vi "Host - Alarm Init (SubVI).vi"(11 "GUI Data in":string[][](array[string])) -> (3 "Alarm Index":T1(array[cluster]))   [LabVIEW 2021]
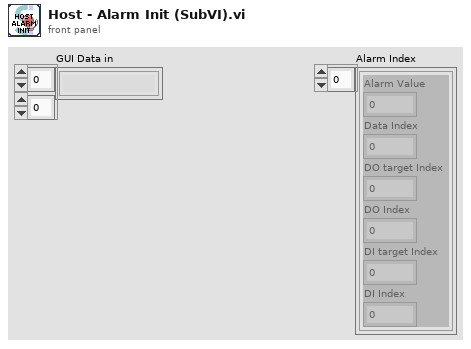
[diagram p1: front panel]
types:
  T1 = cluster{"Alarm Value":dbl, "Data Index":i32, "DO target Index":i32, "DO Index":i32, "DI target Index":i32, "DI Index":i32}[]
  T2 = cluster{"Alarm Value":dbl, "Data Index":i32, "DO target Index":i32, "DO Index":i32, "DI target Index":i32, "DI Index":i32}
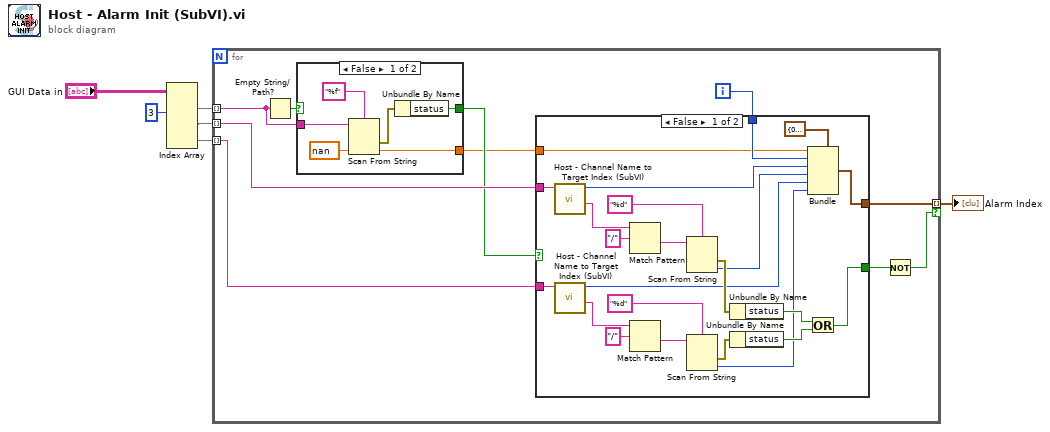
[diagram p0: block diagram]
diagram:
  n1 = Index Array(array="GUI Data in", index (col) #1=3 ("disabled index (col)")) -> (element #1=w4:string[], element #2=w5:string[], element #3=w6:string[])  [unwired: 5 in]
  n2 = for {
    tunnel: w4 -> [w15] mode=indexing
    tunnel: w5 -> [w14] mode=indexing
    tunnel: [w12] -> w1 mode=indexing if=w8
    tunnel: w6 -> [w11] mode=indexing
    i -> [w13]
    n3 = Empty String/Path?(string/path=w15) -> (empty?=w16:bool)
    n4 = case shown="False" w16 {
      selector: w16 -> [_ w47]
      tunnel: w15 -> [w45 _]
      tunnel: [w42 w47] -> w10
      tunnel: [w41 _] -> w7
      frame False {
        n5 = Scan From String(format string="%f", input string=w45, default 1=nan ("default value 1")) -> (error out=w43:errorcluster, output 1=w41:dbl)  [unwired: 2 in, 2 out]
        n6 = Unbundle By Name(w43) -> ("status"=w42:bool)
      }
      frame True {
      }
    }
    n7 = case shown="False" w10 {
      selector: w10 -> [_ w40]
      tunnel: w14 -> [w39 _]
      tunnel: w13 -> [w18 _]
      tunnel: [w34 _] -> w12
      tunnel: w11 -> [w28 _]
      tunnel: [w23 w40] -> w9
      tunnel: w7 -> [w17 _]
      frame False {
        n8 = call "Host - Channel Name to Target Index (SubVI).vi"("Channel In"=w39) -> ("Channel Out"=w35:string, "Target Index"=w19:i32)  [unwired: 8 in, 1 out]
        n9 = call "Host - Channel Name to Target Index (SubVI).vi"("Channel In"=w28) -> ("Channel Out"=w32:string, "Target Index"=w21:i32)  [unwired: 8 in, 1 out]
        n10 = Match Pattern(string=w35, regular expression="/") -> (after substring=w38:string)  [unwired: 1 in, 3 out]
        n11 = Match Pattern(string=w32, regular expression="/") -> (after substring=w29:string)  [unwired: 1 in, 3 out]
        n12 = Scan From String(format string="%d", input string=w38) -> (error out=w27:errorcluster, output 1=w20:i32)  [unwired: 3 in, 2 out]
        n13 = Scan From String(format string="%d", input string=w29) -> (error out=w26:errorcluster, output 1=w22:i32)  [unwired: 3 in, 2 out]
        n14 = Unbundle By Name(w27) -> ("status"=w24:bool)
        n15 = Unbundle By Name(w26) -> ("status"=w25:bool)
        n16 = Bundle(cluster=T2 {"Alarm Value"=0.0, "Data Index"=0, "DO target Index"=0, "DO Index"=0, "DI target Index"=0, "DI Index"=0} ("Alarm Data"), "Alarm Value"=w17, "Data Index"=w18, "DO target Index"=w19, "DO Index"=w20, "DI target Index"=w21, "DI Index"=w22) -> (w34:T2)
        n17 = Or(x=w24, y=w25) -> (x .or. y?=w23:bool)
      }
      frame True {
      }
    }
    n18 = Not(x=w9) -> (.not. x?=w8:bool)
  }
  "Alarm Index" <- w1
